vi "Inline Rx Wait.vi"(8 "error in (no error)":errorcluster, 10 "Dispatcher Interface in":refnum<class "Dispatcher Interface.lvclass">, 11 "Plugin Timing Group in":refnum<class "Plugin Timing.lvclass">) -> (0 "error out":errorcluster, 2 "Dispatcher Interface out":refnum<class "Dispatcher Interface.lvclass">, 3 "Plugin Timing Group out":refnum<class "Plugin Timing.lvclass">)   [LabVIEW 2017, in "DSF Core.lvlib" / "Plugin Timing.lvclass"]
uses:
  Plugin Timing.lvclass
  Interfaces/Dispatcher/Dispatcher Interface.lvclass
  Plugin Timing.lvclass/Plugin Timing.ctl
  Transfer Group Timing.lvclass
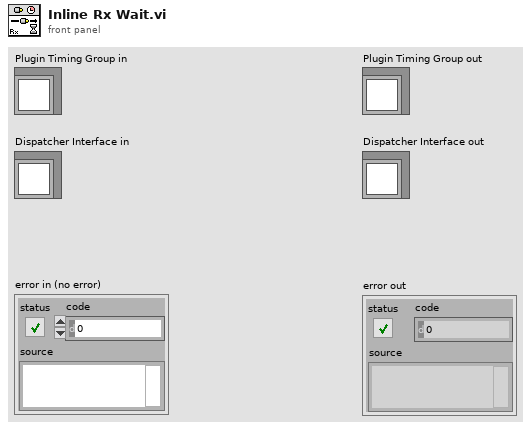
[diagram p1: front panel]
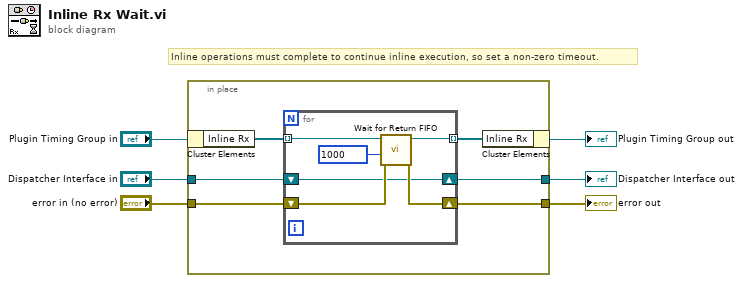
[diagram p0: block diagram]
diagram:
  # "Inline operations must complete to continue inline execution, so set a non-zero timeout."
  n1 = in-place {
    in-place-border: "Dispatcher Interface in" -> [w10]
    in-place-border: [w9] -> w4
    in-place-border: [w8] -> w2
    in-place-border: "error in (no error)" -> [w7]
    n2 = in-place-cluster #1("Plugin Timing Group in") -> ("Inline Rx"=w12:refnum<class "Transfer Group Timing.lvclass">[])
    n3 = for {
      tunnel: w12 -> [w18] mode=indexing
      tunnel: [w14] -> w11 mode=indexing
      shift-right: [w15] -> w9
      shift-left: w10 -> [w15]
      shift-right: [w16] -> w8
      shift-left: w7 -> [w17]
      n4 = call "Wait for Return FIFO.vi"("error in (no error)"=w17, "timeout (0 ms)"=1000, "Transfer Group Timing in"=w18) -> ("error out"=w16:errorcluster, "Transfer Group Timing out"=w14:refnum<class "Transfer Group Timing.lvclass">)  [unwired: 6 in, 1 out]
    }
    n5 = in-place-cluster #1("Inline Rx"=w11) -> (→"Plugin Timing Group out":refnum<class "Plugin Timing.lvclass">)
  }
  "Dispatcher Interface out" <- w4
  "error out" <- w2
